vi "Start Module2.vi"(6 "Show Main VI Diagram on Init (F)":bool, 8 "error in":errorcluster) -> (0 "error out":errorcluster, 1 "Wait for Event Sync?":bool, 2 "FlexiFlowInterface Broadcast Events":T1, 3 "Module Was Already Running?":bool)   [LabVIEW 2025, in "FlexiFlowInterface.lvlib"]
doc: "Launches the Module Main.vi.\n_____\nCreated using DQMH Event Scripter 7.0.1.1316."
uses:
  FlexiFlowInterface/FlexiFlowInterface.lvlib
  <vilib>/Utility/error.llb/Error Cluster From Error Code.vi
  <vilib>/ErrorRing/Error Ring.xnode
  <vilib>/Delacor/Delacor QMH/Libraries/Module Admin_class/Delacor_lib_QMH_Module Admin.lvclass
  FlexiFlowInterface/Did Init Argument--cluster.ctl
  FlexiFlowInterface/Status Updated Argument--cluster.ctl
  FlexiFlowInterface/Error Reported Argument--cluster.ctl
  FlexiFlowInterface/Stop Argument--cluster.ctl
  FlexiFlowInterface/Get Module Execution Status Argument--cluster.ctl
  phlair-shared-libraries/Modbus Flexi-Flow API/Control Function Values--enum.ctl
  phlair-shared-libraries/Modbus Flexi-Flow API/Bronkhorst Flexi-Flow ModbusTCP API.lvlib
  phlair-shared-libraries/Modbus Flexi-Flow API/Control Mode--enum.ctl
  FlexiFlowInterface/Modbus Flexi-Flow Controls--cluster.ctl
  FlexiFlowInterface/Modbus Flexi-Flow Measure State--cluster.ctl
  <vilib>/Plasmionique/MB Master/MB_Master_TCP/MB_Master_TCP.lvclass
  FlexiFlowInterface/Device Type--enum.ctl
  FlexiFlowInterface/Modbus Flexi-Flow State--cluster.ctl
  FlexiFlowInterface/Broadcast Device States Argument--cluster.ctl
  FlexiFlowInterface/Broadcast State (Data Map) Argument--cluster.ctl
  FlexiFlowInterface/Broadcast Events--cluster.ctl
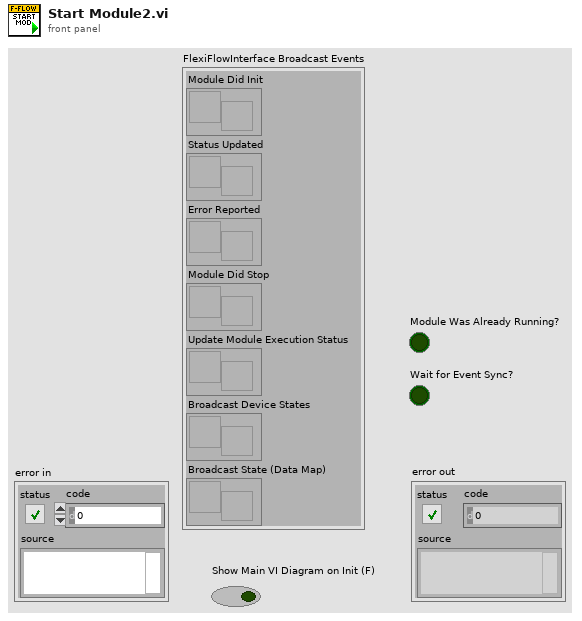
[diagram p1: front panel]
types:
  T1 = typedef "FlexiFlowInterface.lvlib/Broadcast Events--cluster.ctl" = cluster{"Module Did Init":refnum<user-event>, "Status Updated":refnum<user-event>, "Error Reported":refnum<user-event>, "Module Did Stop":refnum<user-event>, "Update Module Execution Status":refnum<user-event>, "Broadcast Device States":refnum<user-event>, "Broadcast State (Data Map)":refnum<user-event>}
  T2 = enum32{"Bad", "Idle", "Run top level", "Running"}
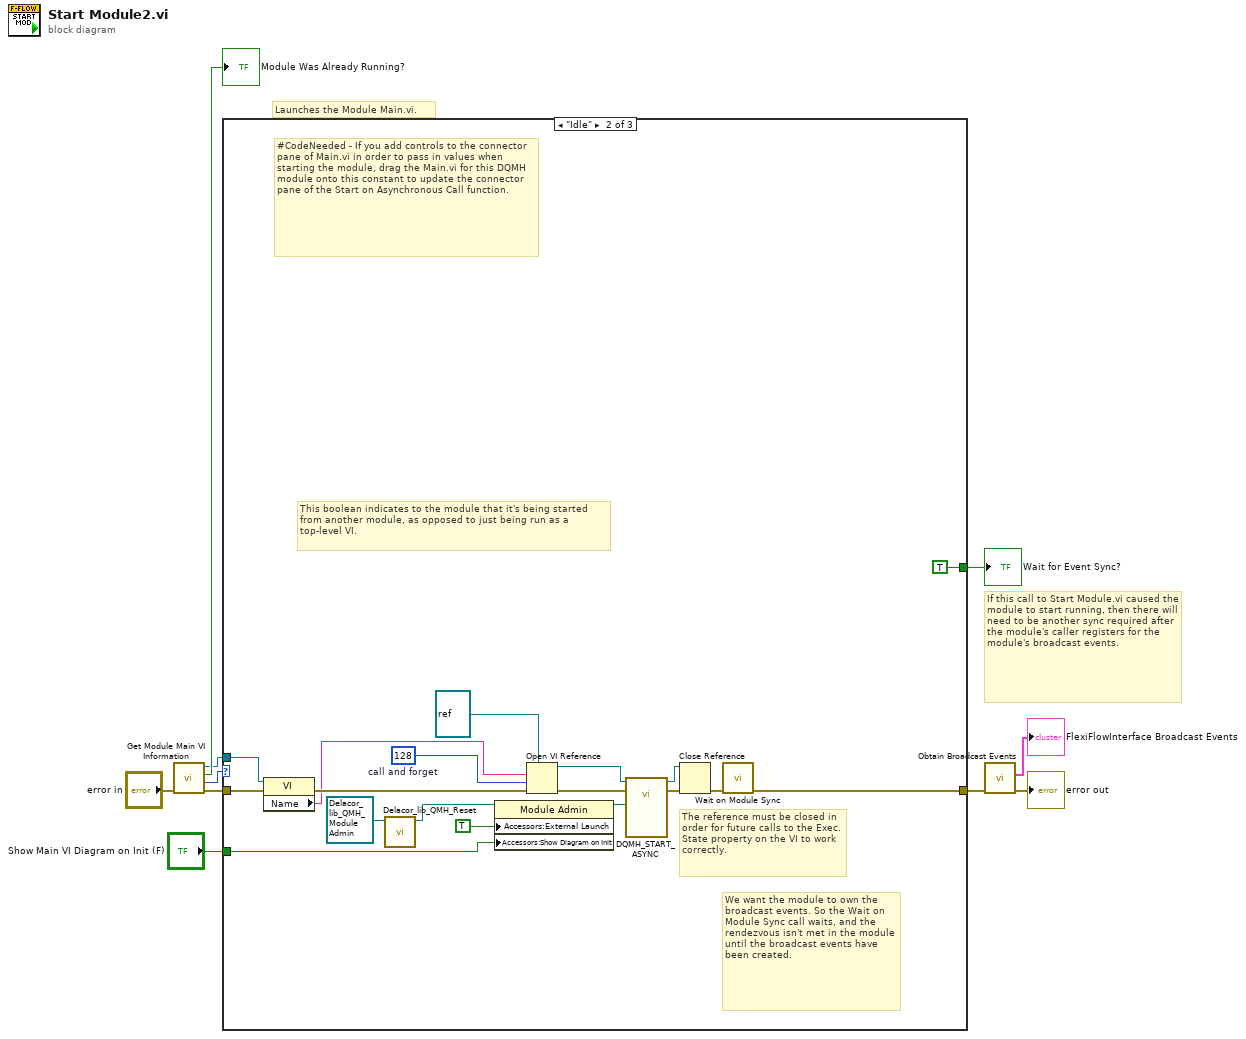
[diagram p0: block diagram]
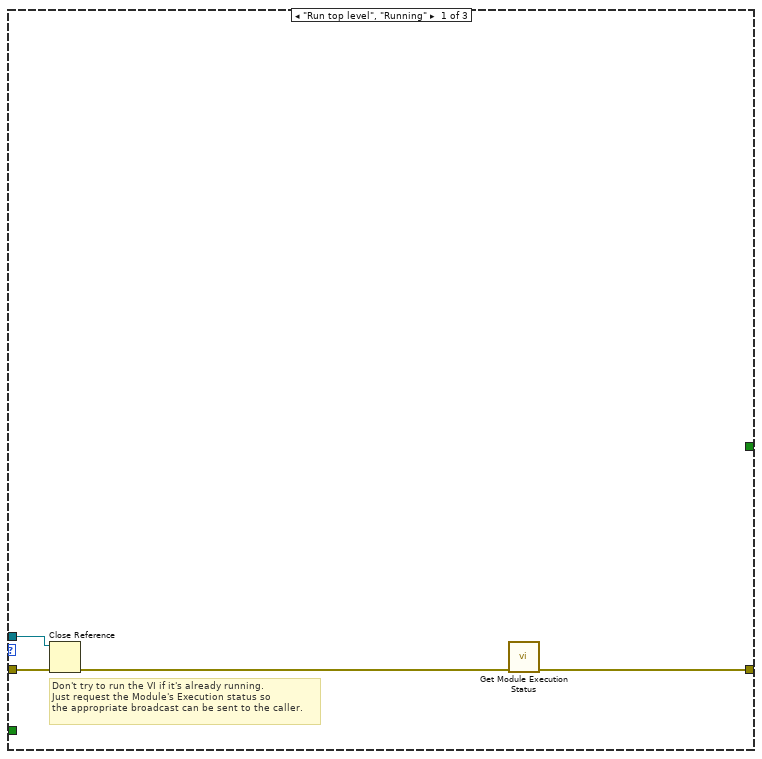
[diagram p2: hidden frame]
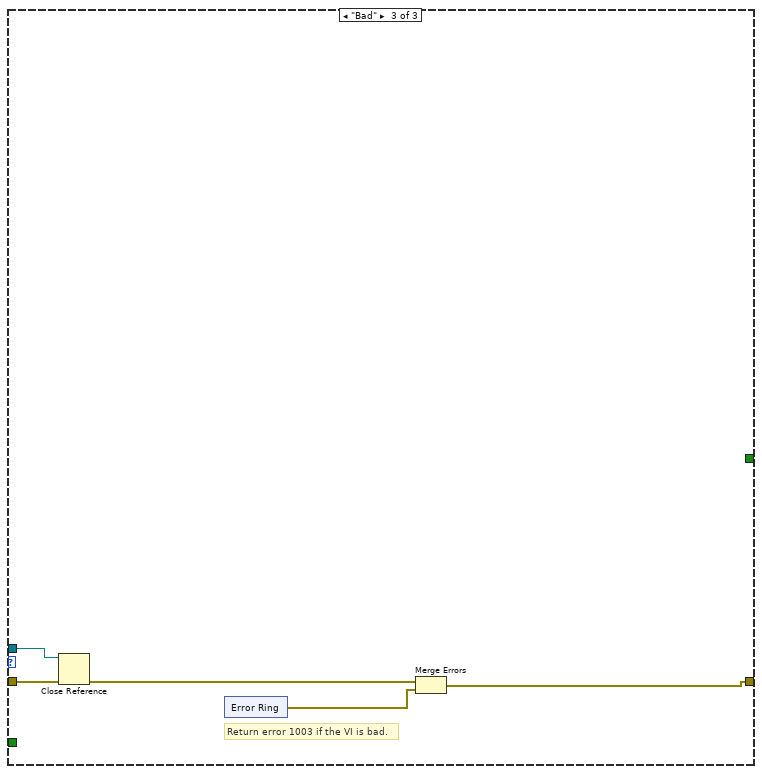
[diagram p3: hidden frame]
diagram:
  # "If this call to Start Module.vi caused the module to start running, then there will need to be another sync required after the module's caller registers for the module's broadcast events."
  # "Launches the Module Main.vi."
  n1 = call "Get Module Main VI Information.vi"("error in (no error)"="error in") -> ("error out"=w8:errorcluster, "Execution State"=w7:T2, "Is Module Running?"=→"Module Was Already Running?":bool, "Module Main VI"=w5:refnum<vi>)  [unwired: 7 in]
  n2 = case shown="\"Idle\"" w7 {
    tunnel: w8 -> [w14 w32 w37]
    tunnel: w5 -> [w13 w27 w36]
    tunnel: [w11 w17 w34] -> w4
    tunnel: [_ TRUE _] -> w10
    tunnel: "Show Main VI Diagram on Init (F)" -> [_ w15 _]
    frame "Run top level", "Running" {
      # "Don't try to run the VI if it's already running.\nJust request the Module's Execution status so\nthe appropriate broadcast can be sent to the caller."
      n3 = Close Reference(reference=w13, error in (no error)=w14) -> (error out=w12:errorcluster)
      n4 = call "Get Module Execution Status.vi"("error in (no error)"=w12) -> ("error out"=w11:errorcluster)  [unwired: 10 in]
    }
    frame "Idle" {
      w24 = 128  # call and forget
      # "#CodeNeeded - If you add controls to the connector pane of Main.vi in order to pass in values when starting the module, drag the Main.vi for this DQMH module onto this constant to update the connector pane of the Start on Asynchronous Call function."
      # "The reference must be closed in order for future calls to the Exec.State property on the VI to work correctly."
      # "We want the module to own the broadcast events. So the Wait on Module Sync call waits, and the rendezvous isn't met in the module until the broadcast events have been created."
      # "This boolean indicates to the module that it's being started from another module, as opposed to just being run as a top-level VI."
      n5 = property class="VI"(reference=w27, error in=w32) -> (error out=w26:errorcluster, "Name"=w19:string)  [unwired: 1 out]
      n6 = call-dynamic "Delacor_lib_QMH_Reset.vi"("Mod Admin in"=refnum<class "Delacor_lib_QMH_Module Admin.lvclass"> refnum) -> ("Mod Admin out"=w30:refnum<class "Delacor_lib_QMH_Module Admin.lvclass">)  [unwired: 9 in, 1 out]
      n7 = property on="DQMH_ADMIN_PROP_NODE" class="Module Admin"(reference=w30, "Accessors:External Launch"=TRUE ("DQMH_EXTERNAL_LAUNCH"), "Accessors:Show Diagram on Init"=w15) -> (reference out=w16:refnum<class "Delacor_lib_QMH_Module Admin.lvclass">)  [unwired: 1 in, 1 out]
      n8 = Open VI Reference(type specifier VI Refnum (for type only)=refnum<vi> refnum ("DQMH_TYPE_SPECIFIER"), vi path=w19, options=w24, error in (no error)=w26) -> (vi reference=w22:refnum<vi>, error out=w23:errorcluster)  [unwired: 2 in]
      n9 = call-by-ref "DQMH_START_ASYNC"(reference=w22, error in=w23, "Module Admin"=w16) -> (reference out=w20:refnum<vi>, error out=w21:errorcluster)  [unwired: 11 in]
      n10 = Close Reference ("DQMH_CLOSE_REF")(reference=w20, error in (no error)=w21) -> (error out=w18:errorcluster)
      n11 = call "Wait on Module Sync.vi"("error in (no error)"=w18) -> ("error out"=w17:errorcluster)  [unwired: 10 in]
    }
    frame "Bad" {
      # "Return error 1003 if the VI is bad."
      n12 = Close Reference(reference=w36, error in (no error)=w37) -> (error out=w35:errorcluster)
      n13 = xnode "Error Ring"() -> ("error out"=w33:errorcluster)
      n14 = Merge Errors(w35, w33) -> (w34:errorcluster)
    }
  }
  "Wait for Event Sync?" <- w10
  n15 = call "Obtain Broadcast Events.vi"("error in (no error)"=w4) -> ("error out"=→"error out":errorcluster, "FlexiFlowInterface Broadcast Events"=→"FlexiFlowInterface Broadcast Events":T1)  [unwired: 9 in]
